vi "reorder array.vi"(8 "Error In":errorcluster, 10 "InArray":u8[](array[numeric]), 11 ".NET (Reference)":refnum<k24>) -> (0 "Error Out":errorcluster, 3 "Array":u8[][](array[numeric]))   [LabVIEW 2018]
doc: "ArrayToVision converts 24/32-bit one-dimensional arrays to a two-dimensional U32 array."
uses:
  C:/Program Files/National Instruments/LabVIEW 2018/instr.lib/IDS/ueye.NET/uEyeDotNet.dll
  instr.lib/IDS/ueye.NET/uEyeDotNet.dll
panel:
  # "Input"
  # "Output"
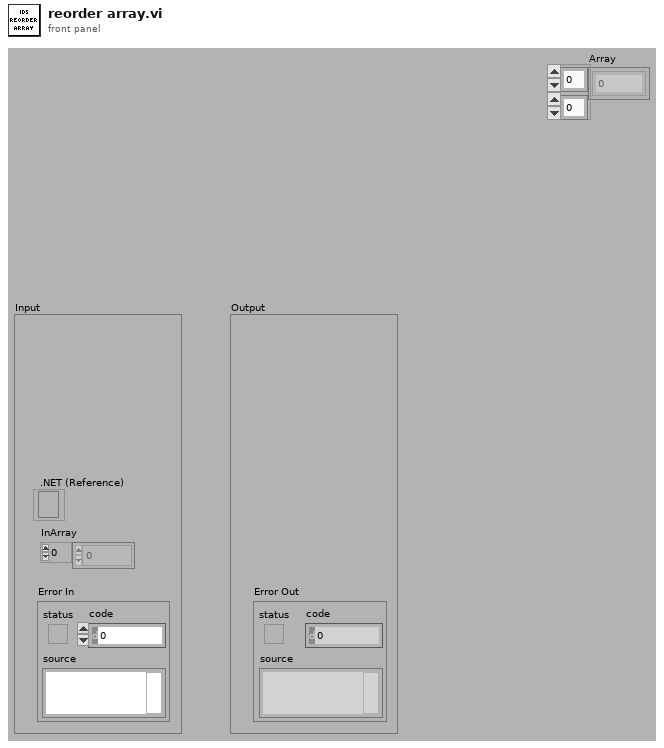
[diagram p1: front panel]
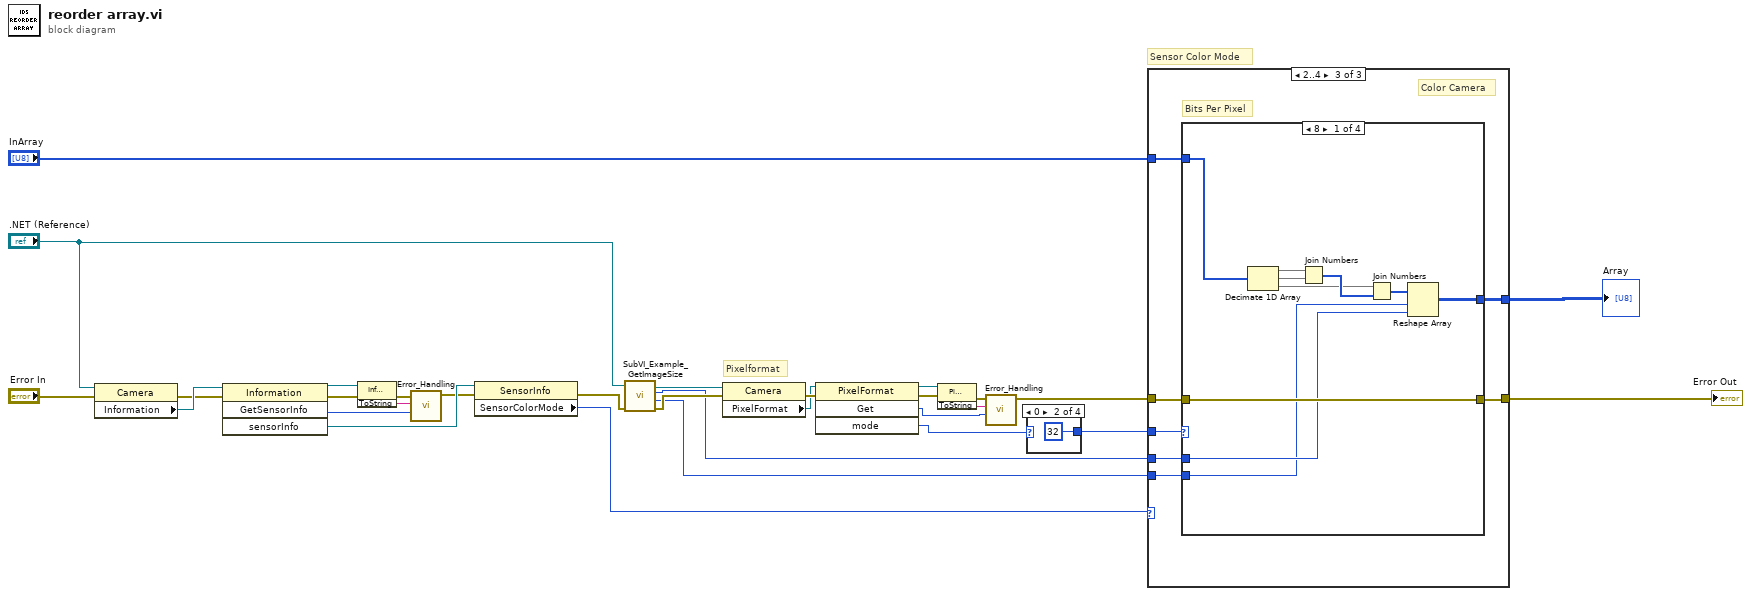
[diagram p0: block diagram]
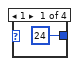
[diagram p2: hidden frame]
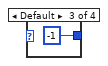
[diagram p3: hidden frame]
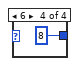
[diagram p4: hidden frame]
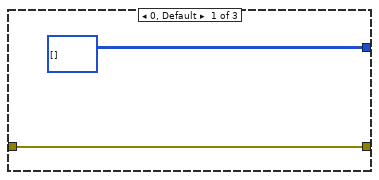
[diagram p5: hidden frame]
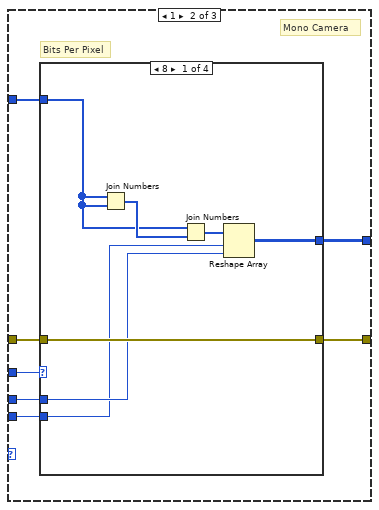
[diagram p6: hidden frame]
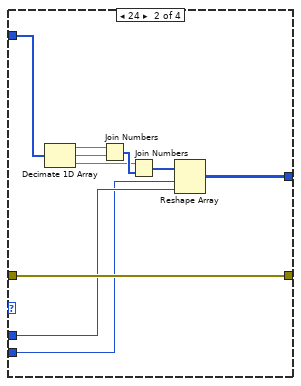
[diagram p7: hidden frame]
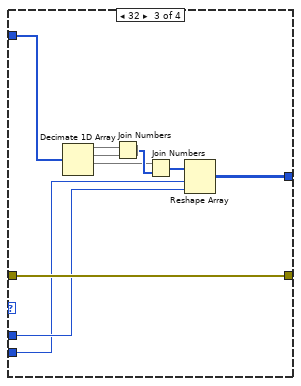
[diagram p8: hidden frame]
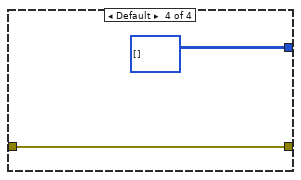
[diagram p9: hidden frame]
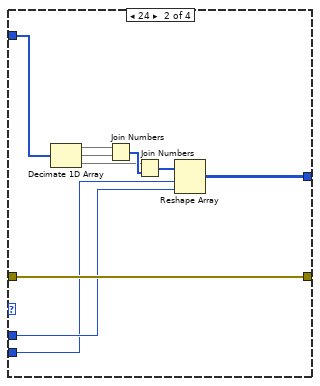
[diagram p10: hidden frame]
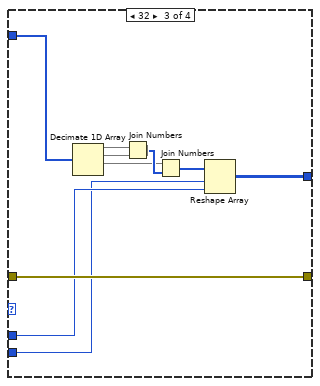
[diagram p11: hidden frame]
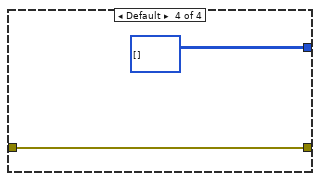
[diagram p12: hidden frame]
diagram:
  # "Sensor Color Mode"
  # "Pixelformat"
  n1 = property on="Eigenschaftsknoten" class="Camera"(reference=".NET (Reference)", error in="Error In") -> (error out=w27:errorcluster, "Information"=w30:refnum<k24>)  [unwired: 1 out]
  n2 = invoke class="Information" method="GetSensorInfo"(reference=w30, error in=w27) -> (reference out=w22:refnum<k24>, error out=w21:errorcluster, "GetSensorInfo"=w20:i32, "sensorInfo"=w29:refnum<k24>)  [unwired: 2 in]
  n3 = invoke class="Information" method="ToString"(reference=w22, error in=w21) -> (error out=w24:errorcluster, "ToString"=w23:string)  [unwired: 1 in, 1 out]
  n4 = call <instrlib>:"Error_Handling.vi"("Error Code"=w20, "Error String"=w23, "Error In"=w24) -> ("Error Out"=w19:errorcluster)  [unwired: 8 in]
  n5 = property class="SensorInfo"(reference=w29, error in=w19) -> (error out=w7:errorcluster, "SensorColorMode"=w28:i32)  [unwired: 1 out]
  n6 = call <instrlib>:"SubVI_Example_GetImageSize.vi"("Error In"=w7, ".NET (Reference)"=".NET (Reference)") -> ("Error Out"=w6:errorcluster, "Height"=w2:i32, "Width"=w3:i32, ".NET (Reference)"=w4:refnum<k24>)  [unwired: 6 in]
  n7 = property class="Camera"(reference=w4, error in=w6) -> (error out=w13:errorcluster, "PixelFormat"=w12:refnum<k24>)  [unwired: 1 out]
  n8 = invoke class="PixelFormat" method="Get"(reference=w12, error in=w13) -> (reference out=w18:refnum<k24>, error out=w17:errorcluster, "Get"=w16:i32, "mode"=w11:i32)  [unwired: 2 in]
  n9 = invoke class="PixelFormat" method="ToString"(reference=w18, error in=w17) -> (error out=w14:errorcluster, "ToString"=w15:string)  [unwired: 1 in, 1 out]
  n10 = call <instrlib>:"Error_Handling.vi"("Error Code"=w16, "Error String"=w15, "Error In"=w14) -> ("Error Out"=w9:errorcluster)  [unwired: 8 in]
  n11 = case shown="0" w11 {
    tunnel: [24 32 -1 8] -> w10
    frame 1 {
    }
    frame 0 {
    }
    frame Default {
    }
    frame 6 {
    }
  }
  n12 = case shown="2..4" w28 {
    tunnel: "InArray" -> [_ w40 w79]
    tunnel: w3 -> [_ w38 w74]
    tunnel: w2 -> [_ w37 w73]
    tunnel: w10 -> [_ w39 w75]
    tunnel: w9 -> [w35 w43 w76]
    tunnel: [w35 w42 w77] -> w8
    tunnel: [u32[][] [] w41 w78] -> w1
    frame 0, Default {
    }
    frame 1 {
      # "Bits Per Pixel"
      # "Mono Camera"
      n13 = case shown="8" w39 {
        tunnel: w40 -> [w46 w55 w64 _]
        tunnel: w37 -> [w44 w51 w61 _]
        tunnel: w38 -> [w45 w52 w62 _]
        tunnel: [w50 w54 w65 u32[][] []] -> w41
        tunnel: w43 -> [w49 w53 w63 w71]
        tunnel: [w49 w53 w63 w71] -> w42
        frame 8 {
          n14 = Join Numbers(hi=w46, lo=w46) -> ((hi.lo)=w48:u16[])
          n15 = Join Numbers(hi=w46, lo=w48) -> ((hi.lo)=w47:u32[])
          n16 = Reshape Array(w47, w44, w45) -> (w50:u32[][])
        }
        frame 24 {
          n17 = Decimate 1D Array(w55) -> (w60:u8[], w59:u8[], w57:u8[])
          n18 = Join Numbers(hi=w59, lo=w60) -> ((hi.lo)=w58:u16[])
          n19 = Join Numbers(hi=w57, lo=w58) -> ((hi.lo)=w56:u32[])
          n20 = Reshape Array(w56, w51, w52) -> (w54:u32[][])
        }
        frame 32 {
          n21 = Decimate 1D Array(w64) -> (w70:u8[], w69:u8[], w67:u8[])  [unwired: 1 out]
          n22 = Join Numbers(hi=w69, lo=w70) -> ((hi.lo)=w68:u16[])
          n23 = Join Numbers(hi=w67, lo=w68) -> ((hi.lo)=w66:u32[])
          n24 = Reshape Array(w66, w61, w62) -> (w65:u32[][])
        }
        frame Default {
        }
      }
    }
    frame 2..4 {
      # "Bits Per Pixel"
      # "Color Camera"
      n25 = case shown="8" w75 {
        tunnel: w79 -> [w81 w94 w103 _]
        tunnel: w73 -> [w86 w90 w100 _]
        tunnel: w74 -> [w87 w91 w101 _]
        tunnel: [w89 w93 w104 u32[][] []] -> w78
        tunnel: w76 -> [w88 w92 w102 w110]
        tunnel: [w88 w92 w102 w110] -> w77
        frame 8 {
          n26 = Decimate 1D Array(w81) -> (w85:u8[], w84:u8[], w82:u8[])
          n27 = Join Numbers(hi=w84, lo=w85) -> ((hi.lo)=w83:u16[])
          n28 = Join Numbers(hi=w82, lo=w83) -> ((hi.lo)=w80:u32[])
          n29 = Reshape Array(w80, w86, w87) -> (w89:u32[][])
        }
        frame 24 {
          n30 = Decimate 1D Array(w94) -> (w99:u8[], w98:u8[], w96:u8[])
          n31 = Join Numbers(hi=w98, lo=w99) -> ((hi.lo)=w97:u16[])
          n32 = Join Numbers(hi=w96, lo=w97) -> ((hi.lo)=w95:u32[])
          n33 = Reshape Array(w95, w90, w91) -> (w93:u32[][])
        }
        frame 32 {
          n34 = Decimate 1D Array(w103) -> (w109:u8[], w108:u8[], w106:u8[])  [unwired: 1 out]
          n35 = Join Numbers(hi=w108, lo=w109) -> ((hi.lo)=w107:u16[])
          n36 = Join Numbers(hi=w106, lo=w107) -> ((hi.lo)=w105:u32[])
          n37 = Reshape Array(w105, w100, w101) -> (w104:u32[][])
        }
        frame Default {
        }
      }
    }
  }
  "Error Out" <- w8
  "Array" <- w1
